vi "FindTag2__slk_tc.vi"(0 "tree control in":refnum<class "TreeControl.lvclass">, 5 "input text":string, 9 "parent tag":string, 11 "error in (no error)":errorcluster, 12 "column # (0)":i32) -> (4 "tree control out":refnum<class "TreeControl.lvclass">, 6 "duplicated text":string, 10 "tags":string[](array[string]), 15 "error out":errorcluster)   [LabVIEW 2020, in "TreeControl.lvclass"]
doc: "Searches the tree for tags whose text matches the Input text."
uses:
  Library/TreeControl.lvclass
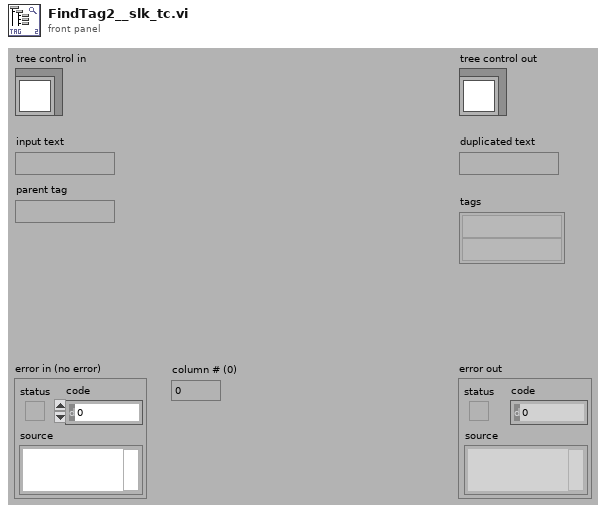
[diagram p1: front panel]
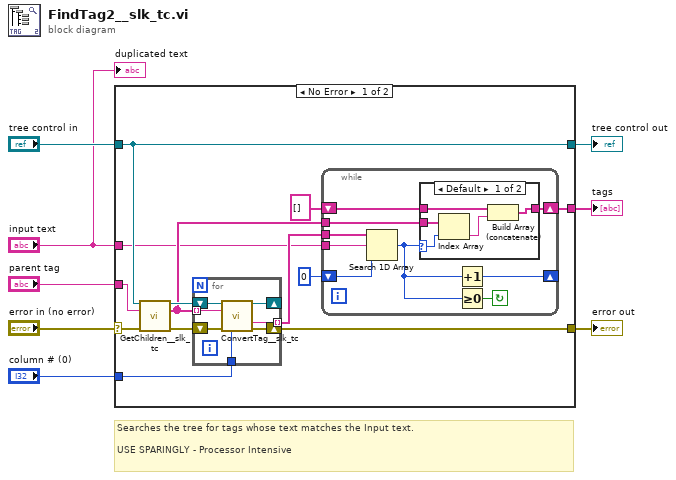
[diagram p0: block diagram]
diagram:
  # "Searches the tree for tags whose text matches the Input text.\n \nUSE SPARINGLY - Processor Intensive"
  n1 = case shown="No Error" "error in (no error)" {
    selector: "error in (no error)" -> [w17 w45]
    tunnel: [w10 w45] -> w7
    tunnel: [w20 w44] -> w5
    tunnel: "tree control in" -> [w20 w44]
    tunnel: "input text" -> [w12 _]
    tunnel: "column # (0)" -> [w18 _]
    tunnel: [w11 _] -> w3
    tunnel: "parent tag" -> [w9 _]
    frame No Error {
      n2 = call "GetChildren__slk_tc.vi"("tree control in"=w20, "parent tag (\"\")"=w9, "error in (no error)"=w17) -> ("tree control out"=w21:refnum<class "TreeControl.lvclass">, "children tags"=w13:string[], "error out"=w19:errorcluster)  [unwired: 1 in, 9 out]
      n3 = for {
        shift-right: [w41] -> _
        shift-left: w21 -> [w43]
        tunnel: w13 -> [w40] mode=indexing
        shift-right: [w39] -> w10
        shift-left: w19 -> [w42]
        tunnel: [w38] -> w14 mode=indexing
        tunnel: w18 -> [w37]
        n4 = call "ConvertTag__slk_tc.vi"("tree control in"=w43, "input tag (current tag)"=w40, "error in (no error)"=w42, "column # (0)"=w37) -> ("tree control out"=w41:refnum<class "TreeControl.lvclass">, "text"=w38:string, "error out"=w39:errorcluster)  [unwired: 9 out]
      }
      n5 = while {
        tunnel: w14 -> [w30]
        tunnel: w12 -> [w29]
        shift-right: [w27] -> _
        shift-left: 0 ("Start Index (0)") -> [w28]
        shift-right: [w24] -> w11
        shift-left: string[] [] ("Tags") -> [w25]
        tunnel: w13 -> [w22]
        stop <- w23 continue-if-true
        n6 = Search 1D Array(1D array=w30, element=w29, start index (0)=w28) -> (index of element=w26:i32)
        n7 = case shown="Default" w26 {
          selector: w26 -> [w35 _]
          tunnel: w25 -> [w34 w36]
          tunnel: [w33 w36] -> w24
          tunnel: w22 -> [w31 _]
          frame Default {
            n8 = Index Array(array=w31, index=w35) -> (element=w32:string)
            n9 = Build Array (concatenate)(w34, w32) -> (w33:string[])
          }
          frame -1 {
          }
        }
        n10 = Increment(x=w26) -> (x+1=w27:i32)
        n11 = Greater Or Equal To 0?(x=w26) -> (x >= 0?=w23:bool)
      }
    }
    frame Error {
    }
  }
  "error out" <- w7
  "tree control out" <- w5
  "tags" <- w3
  "duplicated text" <- "input text"
